vi "UHR-Fleezers Control (host) - 10.8.vi"() -> ()   [LabVIEW 2014] (continued)
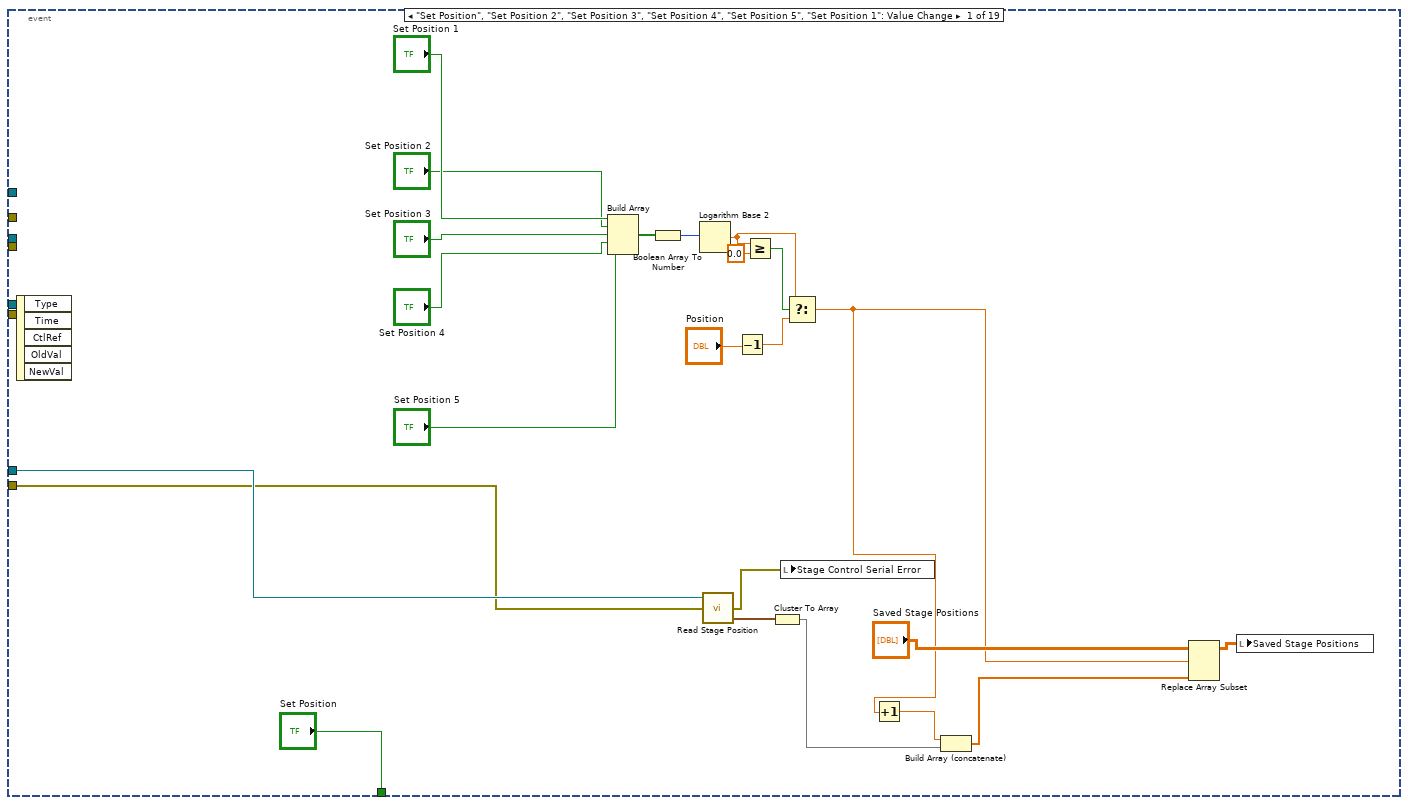
[diagram p2: hidden frame]
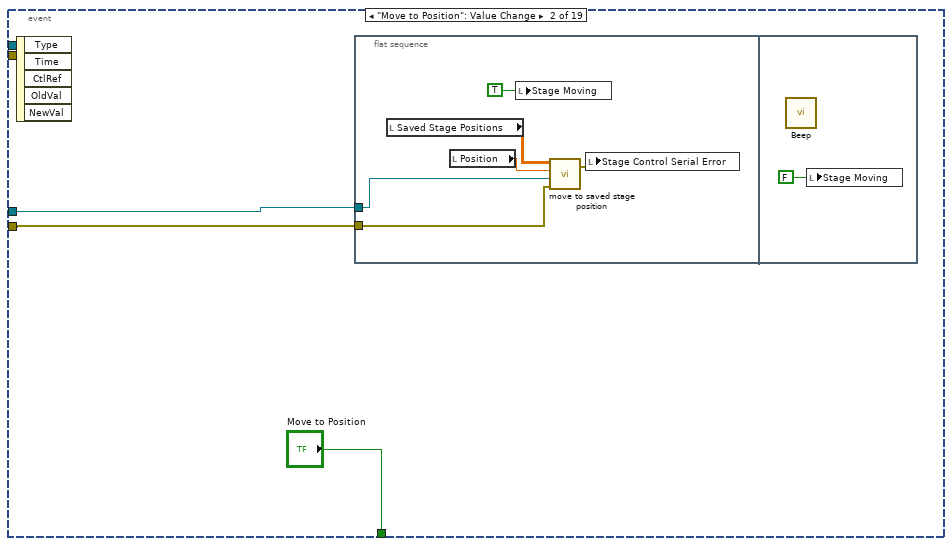
[diagram p3: hidden frame]
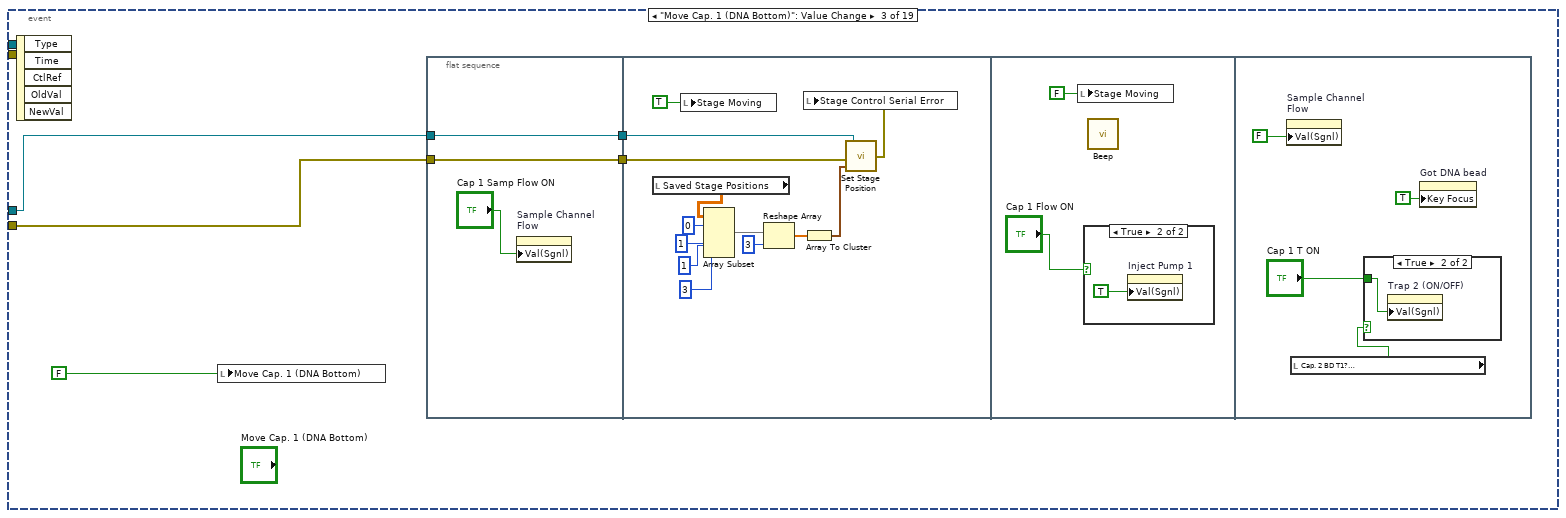
[diagram p4: hidden frame]
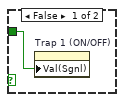
[diagram p6: hidden frame]
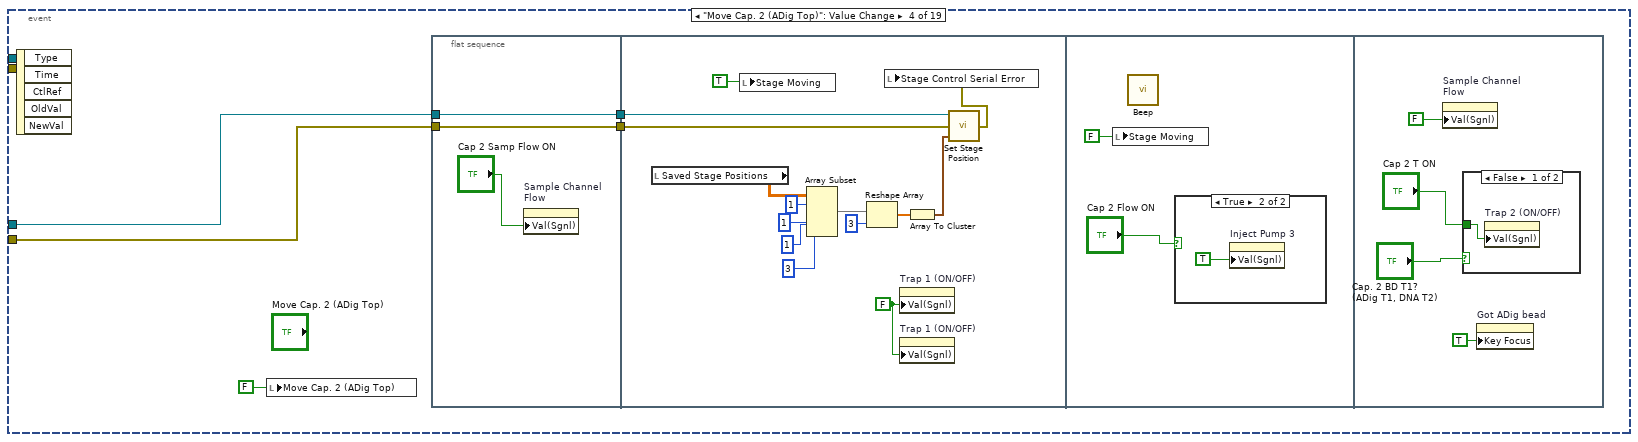
[diagram p7: hidden frame]
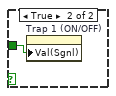
[diagram p9: hidden frame]
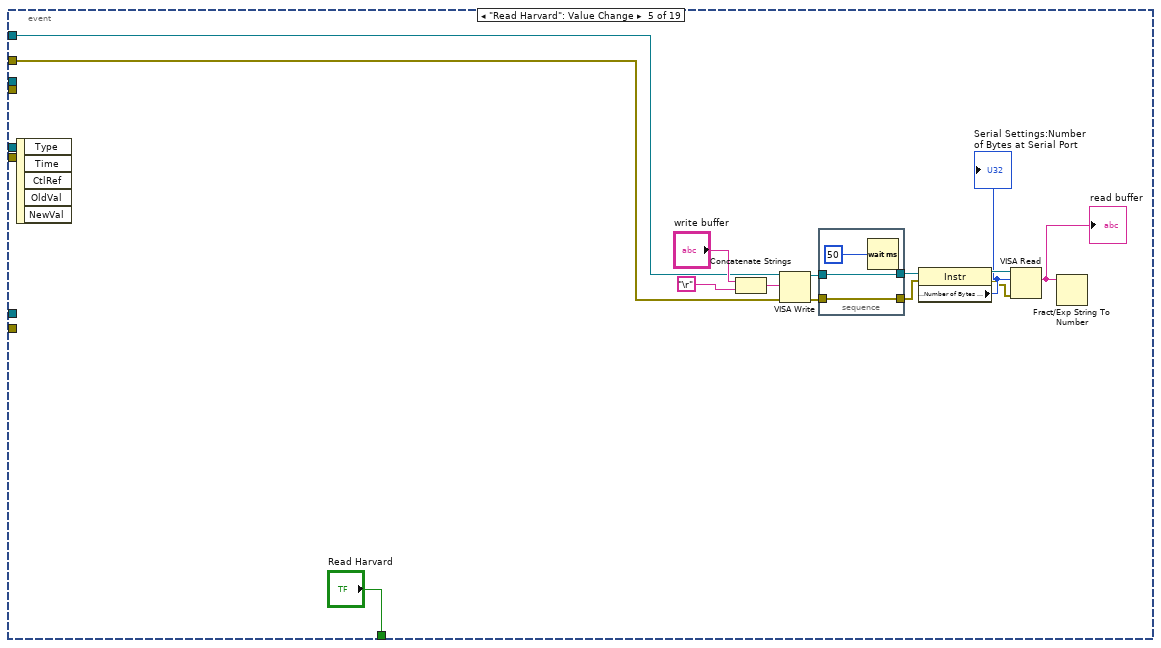
[diagram p10: hidden frame]
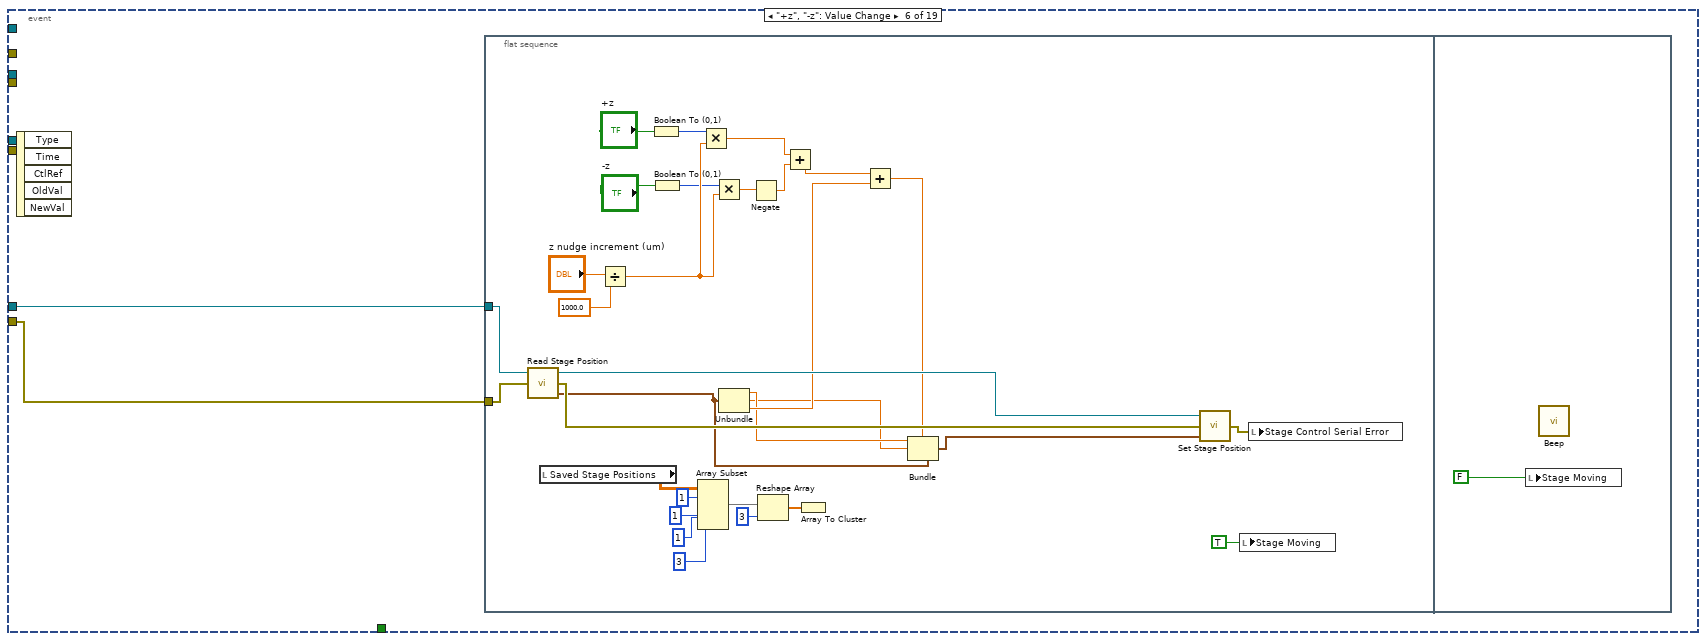
[diagram p11: hidden frame]
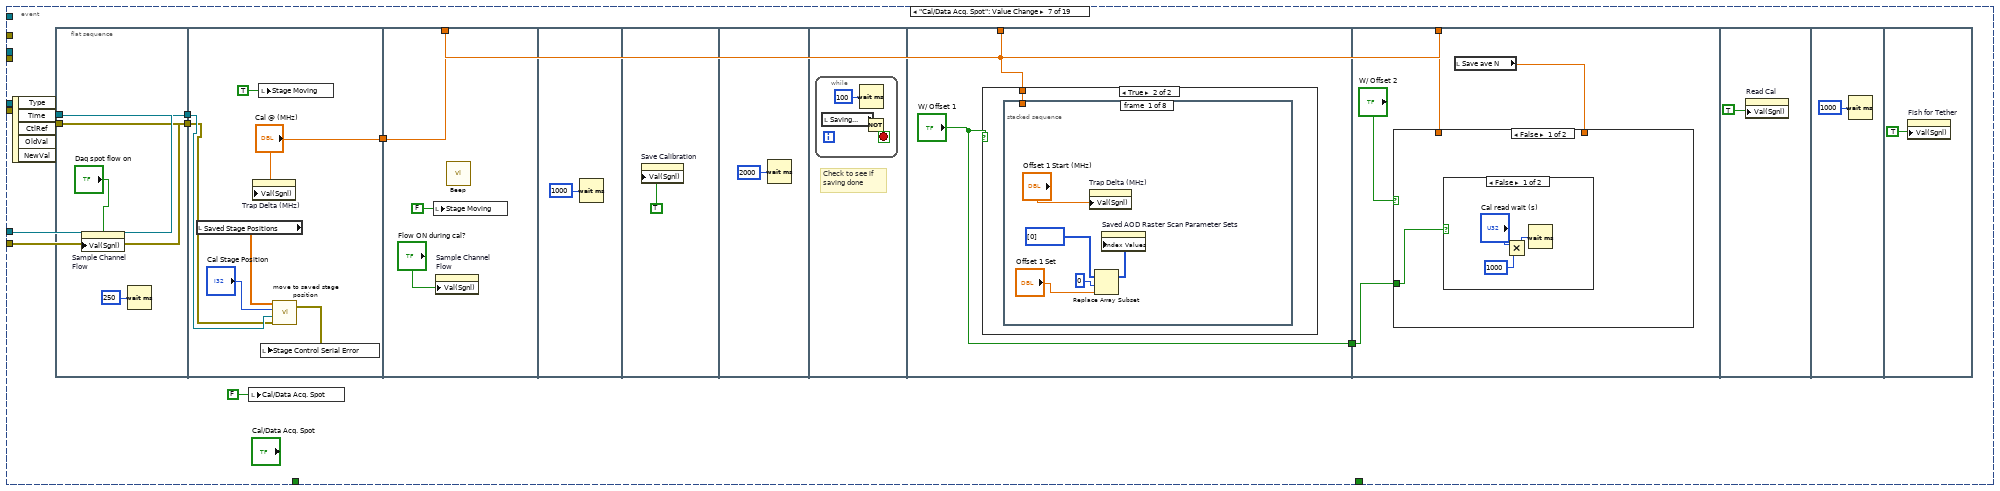
[diagram p12: hidden frame]
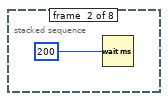
[diagram p14: hidden frame]
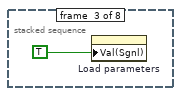
[diagram p15: hidden frame]
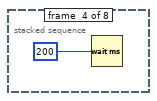
[diagram p16: hidden frame]
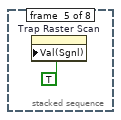
[diagram p17: hidden frame]
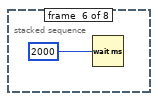
[diagram p18: hidden frame]
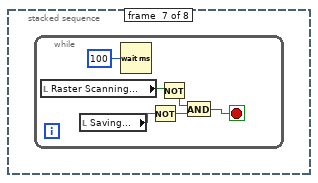
[diagram p19: hidden frame]
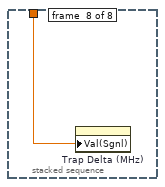
[diagram p20: hidden frame]
            n2757 = Open/Create/Replace File(file path (use dialog)=w4362, operation (0:open)=T25."create", access (0:read/write)=enum16{"read/write", "read-only", "write-only"}."write-only") -> (refnum out=w4400:refnum<file>)  [unwired: 1 in, 4 out]
            n2758 = local write "Saving..."(TRUE ("Saving...")) -> ()
            n2759 = To Double Precision Float(number=w4387) -> (double precision float=w4385:dbl)
            n2760 = String Length(string="Comment (data description)") -> (length=w4383:i32)
            n2761 = To Double Precision Float(number=w4383) -> (double precision float=w4382:dbl)
            n2762 = Deny Access(7:w4400) -> (3:w4399:refnum<file>)  [unwired: 1 in, 2 out]
            n2763 = Build Array (concatenate)(w4385, w4386, w4382) -> (w4384:dbl[])
            n2764 = case "If fluorescence data to be saved" shown="True" w4373 {
              tunnel: w4362 -> [_ w4452]
              tunnel: [refnum<k0> refnum w4432] -> w4374
              frame False {
              }
              frame True {
                w4431 = 0.0
                n2765 = local read "APD Integration Time (s)"() -> (w4437:dbl)
                n2766 = local read "N APD Samp/step"() -> (w4430:dbl)
                n2767 = Path To String(path=w4452) -> (string=w4451:string)
                n2768 = String Length(string=w4451) -> (length=w4450:i32)
                n2769 = Subtract(x=w4450, y=4) -> (x-y=w4448:i32)
                n2770 = String Subset(string=w4451, length (rest)=w4448) -> (substring=w4447:string)  [unwired: 1 out]
                n2771 = Build Array(w4437, w4430, w4431, w4431, w4431, w4431, w4431, w4431) -> (w4434:dbl[])
                n2772 = Concatenate Strings(w4447, "_fl.dat" ("string")) -> (w4445:string)
                n2773 = Array Size(array=w4434) -> (size(s)=w4436:i32)
                n2774 = String To Path(string=w4445) -> (path=w4441:path)
                n2775 = Open/Create/Replace File(file path (use dialog)=w4441, operation (0:open)=T25."create", access (0:read/write)=enum16{"read/write", "read-only", "write-only"}."write-only") -> (refnum out=w4442:refnum<file>)  [unwired: 1 in, 4 out]
                n2776 = Deny Access(7:w4442) -> (3:w4438:refnum<file>)  [unwired: 1 in, 2 out]
                n2777 = To Double Precision Float(number=w4436) -> (double precision float=w4435:dbl)
                n2778 = Build Array (concatenate)(w4435, w4434) -> (w4433:dbl[])
                n2779 = Write to Binary File(file (use dialog)=w4438, data=w4433, 5:FALSE ("prepend array or string size? (T)"), 9:T24."big-endian, network order" ("byte order (0:big-endian, network order)")) -> (refnum out=w4432:refnum<file>)  [unwired: 1 in, 3 out]
              }
            }
            n2780 = case shown="True" w4360 {
              tunnel: w4362 -> [_ w4414]
              tunnel: [refnum<k0> refnum w4413] -> w4361
              frame False {
              }
              frame True {
                w4409 = 0.0 ("element")
                n2781 = Path To String(path=w4414) -> (string=w4428:string)
                n2782 = Build Array(w4409, w4409, w4409, w4409, w4409, w4409, w4409, w4409) -> (w4410:dbl[])
                n2783 = String Length(string=w4428) -> (length=w4427:i32)
                n2784 = Subtract(x=w4427, y=4) -> (x-y=w4425:i32)
                n2785 = Array Size(array=w4410) -> (size(s)=w4412:i32)
                n2786 = String Subset(string=w4428, length (rest)=w4425) -> (substring=w4424:string)  [unwired: 1 out]
                n2787 = To Double Precision Float(number=w4412) -> (double precision float=w4411:dbl)
                n2788 = Concatenate Strings(w4424, "_pos.dat" ("string")) -> (w4422:string)
                n2789 = Build Array (concatenate)(w4411, w4410) -> (w4408:dbl[])
                n2790 = String To Path(string=w4422) -> (path=w4418:path)
                n2791 = Open/Create/Replace File(file path (use dialog)=w4418, operation (0:open)=T25."create", access (0:read/write)=enum16{"read/write", "read-only", "write-only"}."write-only") -> (refnum out=w4419:refnum<file>)  [unwired: 1 in, 4 out]
                n2792 = Deny Access(7:w4419) -> (3:w4415:refnum<file>)  [unwired: 1 in, 2 out]
                n2793 = Write to Binary File(file (use dialog)=w4415, data=w4408, 5:FALSE ("prepend array or string size? (T)"), 9:T24."big-endian, network order" ("byte order (0:big-endian, network order)")) -> (refnum out=w4413:refnum<file>)  [unwired: 1 in, 3 out]
              }
            }
            n2794 = Write to Binary File(file (use dialog)=w4399, data=w4384, 5:w4380, 9:w4378) -> (refnum out=w4381:refnum<file>)  [unwired: 1 in, 3 out]
            n2795 = Write to Binary File(file (use dialog)=w4381, data="Comment (data description)", 5:w4380, 9:w4378) -> (refnum out=w4377:refnum<file>)  [unwired: 1 in, 3 out]
          }
        }
        n2796 = feedback-in #28(w4320) -> ()
        n2797 = feedback-in #29(w4347) -> ()
        n2798 = feedback-in #30(w4319) -> ()
        n2799 = feedback-in #31(w4330) -> ()
        n2800 = feedback-in #32(w4333) -> ()
        n2801 = feedback-in #33(w4346) -> ()
        n2802 = feedback-in #34(w4336) -> ()
      }
      frame #1 {
        n2803 = local read "Saving..."() -> (w4577:bool)
        n2804 = case shown="True" w4577 {
          tunnel: w4581 -> [_ w4591]
          tunnel: w4580 -> [_ w4605]
          tunnel: w4579 -> [_ w4601]
          tunnel: w4578 -> [_ w4600]
          tunnel: w4576 -> [_ w4599]
          tunnel: w4575 -> [_ w4594]
          tunnel: w4574 -> [_ w4593]
          tunnel: w4573 -> [_ w4592]
          tunnel: w4572 -> [_ w4590]
          tunnel: w4571 -> [_ w4588]
          tunnel: w4570 -> [_ w4587]
          tunnel: w4569 -> [_ w4586]
          tunnel: w4568 -> [_ w4585]
          tunnel: w4567 -> [_ w4584]
          tunnel: w4566 -> [_ w4583]
          tunnel: w4565 -> [_ w4582]
          frame False {
          }
          frame True {
            n2805 = Multiply(x=w4591, y=w4590) -> (x*y=→"Time (s)":dbl)
            n2806 = Less Or Equal?(x=w4591, y=w4599) -> (x <= y?=w4603:bool)
            n2807 = Or(x="Stop Saving", y="Abort save 2") -> (x .or. y?=w4595:bool)
            n2808 = Not(x=w4595) -> (.not. x?=w4604:bool)
            n2809 = And(x=w4603, y=w4604) -> (x .and. y?=w4602:bool)
            n2810 = case shown="True" w4602 {
              tunnel: w4605 -> [w4612 w4680]
              tunnel: [0.0 w4683] -> w4598
              tunnel: w4591 -> [_ w4681]
              tunnel: w4599 -> [_ w4682]
              tunnel: w4601 -> [_ w4677]
              tunnel: w4600 -> [_ _]
              tunnel: w4594 -> [w4610 w4670]
              tunnel: w4593 -> [w4609 w4671]
              tunnel: w4592 -> [_ w4669]
              tunnel: w4588 -> [_ w4668]
              tunnel: w4587 -> [_ w4622]
              tunnel: w4586 -> [_ w4661]
              tunnel: w4585 -> [_ w4639]
              tunnel: w4584 -> [w4606 w4620]
              tunnel: w4583 -> [w4607 w4619]
              tunnel: w4582 -> [_ w4616]
              frame False {
                w4608 = FALSE
                n2811 = Close File(refnum=w4612) -> ()  [unwired: 1 in, 2 out]
                n2812 = case shown="True" w4609 {
                  tunnel: w4610 -> [_ w4614]
                  frame False {
                  }
                  frame True {
                    n2813 = Close File(refnum=w4614) -> ()  [unwired: 1 in, 2 out]
                  }
                }
                n2814 = case shown="True" w4606 {
                  tunnel: w4607 -> [_ w4613]
                  frame False {
                  }
                  frame True {
                    n2815 = Close File(refnum=w4613) -> ()  [unwired: 1 in, 2 out]
                  }
                }
                n2816 = local write "Raster Scanning..."(w4608) -> ()
                n2817 = local write "Calibrating Trap..."(w4608) -> ()
                n2818 = call <vilib>:"Beep.vi"() -> ()  [unwired: 3 in, 9 out]
                n2819 = local write "Stop Saving"(w4608) -> ()
                "Saving..." <- w4608
              }
              frame True {
                n2820 = local read "Calibrating Trap..."() -> (w4672:bool)
                n2821 = case "Write fl. data" shown="True" w4671 {
                  tunnel: w4670 -> [_ w4706]
                  tunnel: w4669 -> [_ w4705]
                  frame False {
                  }
                  frame True {
                    n2822 = Write to Binary File(file (use dialog)=w4706, data=w4705, 5:FALSE ("prepend array or string size? (T)"), 9:T24."big-endian, network order" ("byte order (0:big-endian, network order)")) -> ()  [unwired: 1 in, 4 out]
                  }
                }
                n2823 = Greater?(x="Save ave N", y=1.0) -> (0:w4675:bool)
                n2824 = Not(x=w4672) -> (.not. x?=w4674:bool)
                n2825 = And(x=w4674, y=w4675) -> (x .and. y?=w4617:bool)
                n2826 = case shown="True" w4617 {
                  tunnel: w4616 -> [w4686 w4697]
                  tunnel: [w4686 w4689] -> w4615
                  tunnel: "Save ave N" -> [_ w4690]
                  frame False {
                  }
                  frame True {
                    w4687 = 2 ("dimension size")
                    n2827 = Array Size(array=w4697) -> (size(s)=w4691:i32)
                    n2828 = Divide(x=w4691, y=w4687) -> (x/y=w4695:dbl)
                    n2829 = Reshape Array(w4697, w4695, w4687) -> (w4696:u64[][])
                    n2830 = Transpose 2D Array(2D array=w4696) -> (transposed array=w4694:u64[][])
                    n2831 = for {
                      tunnel: w4694 -> [w4699] mode=indexing
                      tunnel: [w4698] -> w4688 mode=indexing
                      tunnel: w4690 -> [w4700]
                      workers-P: _ -> [_]
                      n2832 = call "downsample 1D array - U64.vi"("Ave N"=w4700, "Array In"=w4699) -> ("Array Out"=w4698:u64[])  [unwired: 1 in]
                    }
                    n2833 = Transpose 2D Array(2D array=w4688) -> (transposed array=w4693:u64[][])
                    n2834 = Divide(x=w4691, y=w4690) -> (x/y=w4692:dbl)
                    n2835 = Reshape Array(w4693, w4692) -> (w4689:u64[])
                  }
                }
                n2836 = case shown="False" w4617 {
                  tunnel: w4677 -> [w4709 w4721]
                  tunnel: [w4709 w4713] -> w4673
                  tunnel: "Save ave N" -> [_ w4714]
                  tunnel: w4668 -> [_ w4712]
                  frame False {
                  }
                  frame True {
                    n2837 = Array Size(array=w4721) -> (size(s)=w4715:i32)
                    n2838 = Array Size(array=w4712) -> (size(s)=w4711:i32)
                    n2839 = Divide(x=w4715, y=w4711) -> (x/y=w4719:dbl)
                    n2840 = Reshape Array(w4721, w4719, w4711) -> (w4720:i16[][])
                    n2841 = Transpose 2D Array(2D array=w4720) -> (transposed array=w4718:i16[][])
                    n2842 = for {
                      tunnel: w4718 -> [w4724] mode=indexing
                      tunnel: [w4723] -> w4710 mode=indexing
                      tunnel: w4714 -> [w4722]
                      workers-P: _ -> [_]
                      n2843 = call "downsample 1D array - I16.vi"("Ave N"=w4722, "Array In"=w4724) -> ("Array Out"=w4723:i16[])  [unwired: 1 out]
                    }
                    n2844 = Transpose 2D Array(2D array=w4710) -> (transposed array=w4717:i16[][])
                    n2845 = Divide(x=w4715, y=w4714) -> (x/y=w4716:dbl)
                    n2846 = Reshape Array(w4717, w4716) -> (w4713:i16[])
                  }
                }
                n2847 = Index Array(array=w4639, index=1) -> (element=w4642:waveform(dbl))
                n2848 = Index Array(array=w4639, index=0) -> (element=w4644:waveform(dbl))
                n2849 = Unbundle By Name(w4642) -> ("Y"=w4646:dbl[])
                n2850 = Unbundle By Name(w4644) -> ("Y"=w4654:dbl[])
                n2851 = case "Write trap pos. data" shown="True" w4620 {
                  tunnel: w4619 -> [_ w4702]
                  tunnel: w4615 -> [_ w4701]
                  frame False {
                  }
                  frame True {
                    n2852 = Write to Binary File(file (use dialog)=w4702, data=w4701, 5:FALSE ("prepend array or string size? (T)"), 9:T24."big-endian, network order" ("byte order (0:big-endian, network order)")) -> ()  [unwired: 1 in, 4 out]
                  }
                }
                n2853 = Write to Binary File(file (use dialog)=w4680, data=w4673, 5:FALSE ("prepend array or string size? (T)"), 9:T24."big-endian, network order" ("byte order (0:big-endian, network order)")) -> ()  [unwired: 1 in, 4 out]
                n2854 = feedback #35(w4646) -> (w4648:dbl[])
                n2855 = Build Array (concatenate)(w4648, w4646) -> (w4647:dbl[])
                n2856 = Select(t=w4646, s=w4622, f=w4647) -> (s? t:f=w4632:dbl[])
                n2857 = feedback-in #35(w4632) -> ()
                n2858 = feedback #36(w4654) -> (w4667:dbl[])
                n2859 = Build Array (concatenate)(w4667, w4654) -> (w4666:dbl[])
                n2860 = Select(t=w4654, s=w4622, f=w4666) -> (s? t:f=w4641:dbl[])
                n2861 = feedback-in #36(w4641) -> ()
                n2862 = Divide(x=w4681, y=w4682) -> (x/y=w4684:dbl)
                n2863 = Multiply(x=w4684, y=100.0) -> (x*y=w4683:dbl)
                n2864 = Build Array(w4641, w4632) -> (→"Saved APD":dbl[][])
                n2865 = Array Size(array=w4641) -> (size(s)=w4659:i32)
                n2866 = Unbundle By Name(w4661) -> ("Y"=w4665:dbl[])
                n2867 = Subtract(x=w4659, y="N pts to average") -> (x-y=w4635:i32)
                n2868 = Multiply(x="N pts to average", y=u16 2) -> (x*y=w4636:u16)
                n2869 = Subtract(x=w4659, y=w4636) -> (x-y=w4634:i32)
                n2870 = feedback #37(w4665) -> (w4664:dbl[])
                n2871 = Build Array (concatenate)(w4664, w4665) -> (w4663:dbl[])
                n2872 = Select(t=w4665, s=w4622, f=w4663) -> (s? t:f=w4662:dbl[])
                "Trap Delta Graph" <- w4662
                n2873 = feedback-in #37(w4662) -> ()
                n2874 = Array Subset(array=w4641, index=w4635, length="N pts to average") -> (w4658:dbl[])
                n2875 = Array Subset(array=w4641, index=w4634, length="N pts to average") -> (w4657:dbl[])
                n2876 = Array Subset(array=w4632, index=w4635, length="N pts to average") -> (w4638:dbl[])
                n2877 = Array Subset(array=w4632, index=w4634, length="N pts to average") -> (w4637:dbl[])
                n2878 = call-poly <vilib>:"Mean.vi"("X"=w4658) -> ("mean"=w4656:dbl)  [unwired: 1 out]
                n2879 = call-poly <vilib>:"Mean.vi"("X"=w4638) -> ("mean"=w4631:dbl)  [unwired: 1 out]
                n2880 = call-poly <vilib>:"Mean.vi"("X"=w4657) -> ("mean"=w4655:dbl)  [unwired: 1 out]
                n2881 = call-poly <vilib>:"Mean.vi"("X"=w4637) -> ("mean"=w4630:dbl)  [unwired: 1 out]
                n2882 = Subtract(x=w4631, y=w4630) -> (x-y=w4621:dbl)
                "Delta Fl. 2" <- w4621
                n2883 = Subtract(x=w4656, y=w4655) -> (x-y=w4653:dbl)
                "Delta Fl. 1" <- w4653
                n2884 = Initialize Array(w4653, 1 ("dimension size")) -> (w4650:dbl[])
                n2885 = Initialize Array(w4621, 1 ("dimension size")) -> (w4627:dbl[])
                n2886 = feedback #38(w4650) -> (w4651:dbl[])
                n2887 = Build Array (concatenate)(w4651, w4650) -> (w4649:dbl[])
                n2888 = feedback #39(w4627) -> (w4628:dbl[])
                n2889 = Build Array (concatenate)(w4628, w4627) -> (w4626:dbl[])
                n2890 = Select(t=w4650, s=w4622, f=w4649) -> (s? t:f=w4625:dbl[])
                n2891 = feedback-in #38(w4625) -> ()
                n2892 = Select(t=w4627, s=w4622, f=w4626) -> (s? t:f=w4624:dbl[])
                n2893 = feedback-in #39(w4624) -> ()
                n2894 = Build Array(w4625, w4624) -> (→"Save APD Deriv":dbl[][])
              }
            }
            "Progress" <- w4598
            "Progress 2" <- w4598
          }
        }
      }
    }
    n2895 = Bundle By Name(cluster=w3260, "Green FB Ch 0"=w3259, "Green FB Ch 1"=w3258) -> (w3238:cluster{})
    "Green FB Signals (V)" <- w3238
    n2896 = Unbundle By Name(w3238) -> ("Green FB Ch 2"=→"Green FB Plot")
    n2897 = local read "wait to reset values"() -> (w3329:bool)
    n2898 = Not(x=w3327) -> (.not. x?=w3330:bool)
    n2899 = And(x=w3330, y=w3329) -> (x .and. y?=w3331:bool)
    n2900 = case "Part of MCL raster scanning: returns to initial positions after scan done" shown="True" w3331 {
      tunnel: w3044 -> [w4140 w4147]
      tunnel: [w4140 w4146] -> w3333
      tunnel: w3043 -> [w4139 w4145]
      tunnel: [w4139 w4144] -> w3328
      frame False {
      }
      frame True {
        w4155 = 10.0 ("y")
        w4154 = 32767.0 ("y")
        # "to return scan values\nafter a synchronous \nAOM scan"
        n2901 = local read "AO2"() -> (w4148:dbl)
        n2902 = local read "AO1"() -> (w4149:dbl)
        n2903 = local write "wait to reset values"(FALSE ("wait to reset values")) -> ()
        n2904 = Multiply(x=w4149, y=w4154) -> (x*y=w4151:dbl)
        n2905 = Multiply(x=w4148, y=w4154) -> (x*y=w4153:dbl)
        n2906 = Divide(x=w4151, y=w4155) -> (x/y=w4150:dbl)
        n2907 = Divide(x=w4153, y=w4155) -> (x/y=w4152:dbl)
        n2908 = To Word Integer(number=w4150) -> (16bit integer=w4156:i16)
        n2909 = To Word Integer(number=w4152) -> (16bit integer=w4157:i16)
        n2910 = local read "Total Counts (ticks)"() -> (w4141:u32)
        n2911 = xnode "Read/Write Control"("FPGA VI Reference In"=w4147, "error in"=w4145, "AO1"=w4156, "AO2"=w4157, "MCL count"=w4141) -> ("FPGA VI Reference Out"=w4146:T19, "error out"=w4144:errorcluster)
        n2912 = local read "Scan Range (V)\n(of steps)"() -> (w4142:dbl)
        n2913 = property on="Scan Range (V)\n(of steps)" class="DigNum (strict)"("Val(Sgnl)"=w4142) -> ()  [unwired: 2 in, 2 out]
      }
    }
    n2914 = node-c288() -> ()  [unwired: 2 out]
  }
  n2915 = node-c288(w78) -> ()  [unwired: 1 out]
  n2916 = VISA Close(VISA resource name=w82, error in (no error)=w81) -> (error out=w130:errorcluster)
  n2917 = call <vilib>:"Simple Error Handler.vi"("error in (no error)"=w130) -> ()  [unwired: 1 in, 8 out]
  n2918 = node-c288(w89) -> ()  [unwired: 1 out]
  n2919 = node-c288(w174) -> ()  [unwired: 1 out]
  n2920 = flat-sequence {
    tunnel: w268 -> [w4728]
    tunnel: w270 -> [w4729]
    tunnel: [w4727] -> w249
    tunnel: [w4726] -> w248
    tunnel: w230 -> [_]
    tunnel: w182 -> [_]
    tunnel: w95 -> [_]
    tunnel: w249 -> [w4730]
    tunnel: w248 -> [w4731]
    frame #0 {
      w4725 = FALSE ("AI to FIFO")
      n2921 = xnode "Read/Write Control"("FPGA VI Reference In"=w4729, "error in"=w4728, "AI to FIFO"=w4725, "APD to FIFO"=w4725) -> ("FPGA VI Reference Out"=w4727:T19, "error out"=w4726:errorcluster)
    }
    frame #1 {
      n2922 = xnode "Close FPGA VI Reference"("FPGA VI Reference In"=w4730, "error in"=w4731) -> ("error out"=→"error out":errorcluster)
    }
  }
